vi "Acquire multiple shots.vi"(7 "DAQ":T1={"Data"={"Live"={"t0"=timestamp(0 s since 1904-01-01), "dt"=1.0, "Y"=[]}, "Accumulated"={"t0"=timestamp(0 s since 1904-01-01), "dt"=1.0, "Y"=[]}, "Averaged"={"t0"=timestamp(0 s since 1904-01-01), "dt"=1.0, "Y"=[]}, "data array"=[], "live time array"=[], "Live (decimated)"={"t0"=timestamp(0 s since 1904-01-01), "dt"=1.0, "Y"=[]}}, "Config"={"Input Config"=0, "Card"=enum."USB-6211", "100% Reflectance Standard (V)"=0.0, "Input Channel"="", "Average number of points"=0.0, "Trigger Level (V)"=0.0, "Rate (Hz)"=0, "End Time (s)"=0.0}, "Indicators"={"Final number of points"=0.0, "Number of samples"=0.0, "dt"=0.0, "Shots"=10, "Shot counter"=10, "Test counter"=10, "Background level (V)"=0.0, "DAQ task"="", "timestamp of data"=timestamp(0 s since 1904-01-01), "Test Type"=enum."A-Test"}} {"Config"."Input Config" items=["default"=-1, "RSE"=10083, "NRSE"=10078, "Differential"=10106, "Pseudodifferential"=12529]}, 8 "error in (no error)":errorcluster) -> (0 "error out":errorcluster, 5 "DAQ out":T1={"Data"={"Live"={"t0"=timestamp(0 s since 1904-01-01), "dt"=1.0, "Y"=[]}, "Accumulated"={"t0"=timestamp(0 s since 1904-01-01), "dt"=1.0, "Y"=[]}, "Averaged"={"t0"=timestamp(0 s since 1904-01-01), "dt"=1.0, "Y"=[]}, "data array"=[], "live time array"=[], "Live (decimated)"={"t0"=timestamp(0 s since 1904-01-01), "dt"=1.0, "Y"=[]}}, "Config"={"Input Config"=0, "Card"=enum."USB-6211", "100% Reflectance Standard (V)"=0.0, "Input Channel"="", "Average number of points"=0.0, "Trigger Level (V)"=0.0, "Rate (Hz)"=0, "End Time (s)"=0.0}, "Indicators"={"Final number of points"=0.0, "Number of samples"=0.0, "dt"=0.0, "Shots"=10, "Shot counter"=10, "Test counter"=10, "Background level (V)"=0.0, "DAQ task"="", "timestamp of data"=timestamp(0 s since 1904-01-01), "Test Type"=enum."A-Test"}} {"Config"."Input Config" items=["default"=-1, "RSE"=10083, "NRSE"=10078, "Differential"=10106, "Pseudodifferential"=12529]})   [LabVIEW 2017, in "DAQ.lvlib"]
uses:
  DAQ.lvlib
  Controls/Params.ctl
  Controls/DAQ Config.ctl
  Controls/DAQ Indicators.ctl
  System Control/CTLs/Test Type.ctl
  <vilib>/DAQmx/read.llb/DAQmx Read (Analog Wfm 1Chan NSamp).vi
  <vilib>/DAQmx/miscellaneous.llb/DAQmx Fill In Error Info.vi
  System Control/Main controller.lvlib
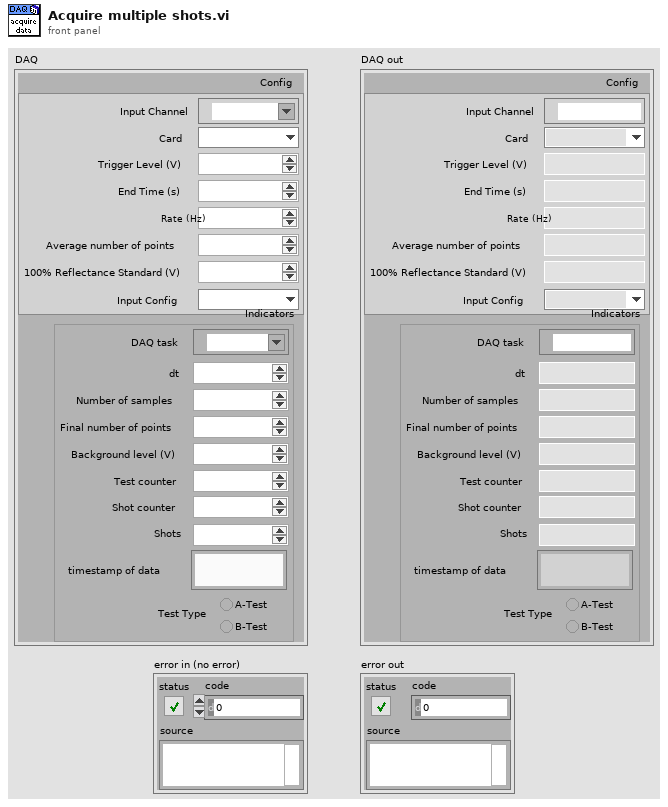
[diagram p1: front panel]
types:
  T1 = typedef "DAQ.lvlib/Params.ctl" = cluster{"Data":cluster{"Live":waveform(dbl), "Accumulated":waveform(dbl), "Averaged":waveform(dbl), "data array":dbl[], "live time array":dbl[], "Live (decimated)":waveform(dbl)}, "Config":T2, "Indicators":T3}
  T2 = typedef "DAQ.lvlib/DAQ Config.ctl" = cluster{"Input Config":i32, "Card":enum16{"USB-6211", "USB-6251", "USB-6361"}, "100% Reflectance Standard (V)":dbl, "Input Channel":tag, "Average number of points":dbl, "Trigger Level (V)":dbl, "Rate (Hz)":i32, "End Time (s)":dbl}
  T3 = typedef "DAQ.lvlib/DAQ Indicators.ctl" = cluster{"Final number of points":dbl, "Number of samples":dbl, "dt":dbl, "Shots":i32, "Shot counter":i32, "Test counter":i32, "Background level (V)":dbl, "DAQ task":refnum<k21>, "timestamp of data":timestamp, "Test Type":T4}
  T4 = typedef "Main controller.lvlib/Test Type.ctl" = enum32{"A-Test", "B-Test"}
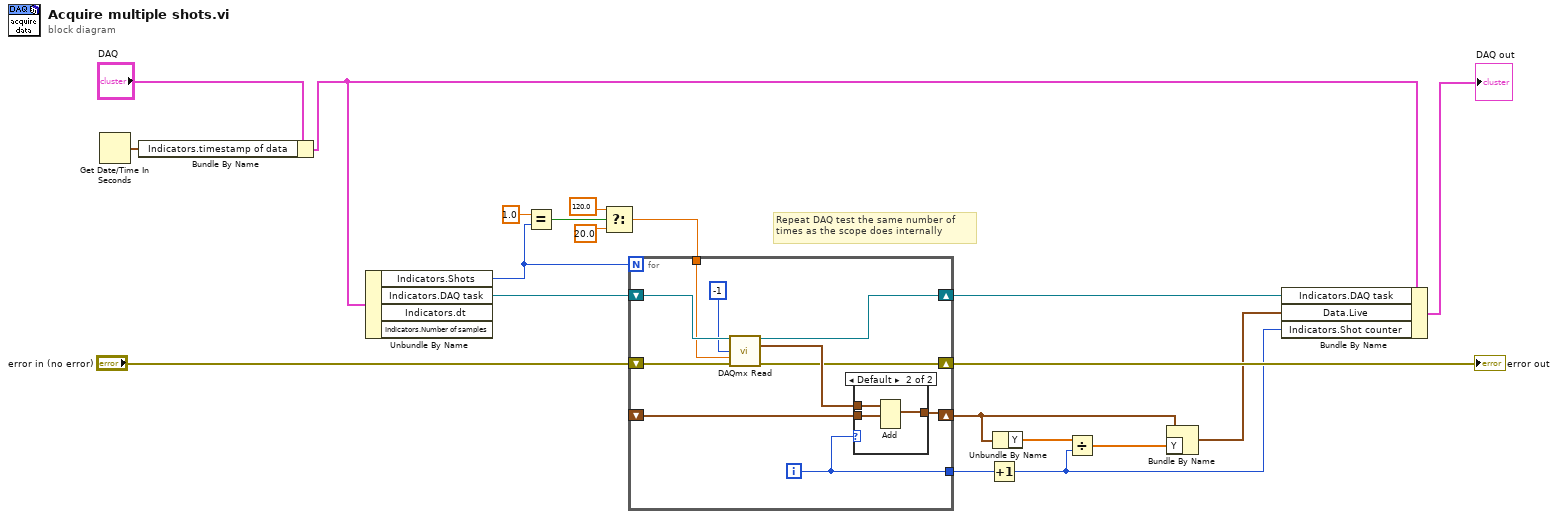
[diagram p0: block diagram]
diagram:
  # "Repeat DAQ test the same number of \ntimes as the scope does internally"
  n1 = Get Date/Time In Seconds() -> (seconds since 1Jan1904=w6:timestamp)
  n2 = Bundle By Name(cluster="DAQ", "Indicators.timestamp of data"=w6) -> (w2:T1)
  n3 = Unbundle By Name(w2) -> ("Indicators.Shots"=w13:i32, "Indicators.DAQ task"=w12:refnum<k21>)  [unwired: 2 out]
  n4 = Equal?(x=1.0 ("y"), y=w13) -> (x = y?=w17:bool)
  n5 = Select(t=120.0 ("timeout"), s=w17, f=20.0 ("timeout")) -> (s? t:f=w14:dbl)
  n6 = for {
    N: w13 -> [_]
    shift-right: [w26] -> w9
    shift-left: _ -> [w30]
    shift-right: [w22] -> w20
    shift-left: "error in (no error)" -> [w28]
    shift-right: [w29] -> w11
    shift-left: w12 -> [w27]
    tunnel: w14 -> [w23]
    tunnel: [w21] -> w8
    i -> [w21]
    n7 = call-poly <vilib>:"DAQmx Read.vi"("task/channels in"=w27, "number of samples per channel"=-1, "timeout"=w23, "error in"=w28) -> ("task out"=w29:refnum<k21>, "data"=w25:waveform(dbl), "error out"=w22:errorcluster)  [unwired: 9 in]
    n8 = case shown="Default" w21 {
      tunnel: w30 -> [_ w34]
      tunnel: [w31 w33] -> w26
      tunnel: w25 -> [w31 w32]
      frame 0 {
      }
      frame Default {
        n9 = Add(1:w34, 2:w32) -> (0:w33:waveform(dbl))  [unwired: 1 in, 1 out]
      }
    }
  }
  "error out" <- w20
  n10 = Increment(x=w8) -> (x+1=w7:i32)
  n11 = Unbundle By Name(w9) -> ("Y"=w3:dbl[])
  n12 = Divide(x=w3, y=w7) -> (x/y=w1:dbl[])
  n13 = Bundle By Name(cluster=w9, "Y"=w1) -> (w4:waveform(dbl))
  n14 = Bundle By Name(cluster=w2, "Indicators.DAQ task"=w11, "Data.Live"=w4, "Indicators.Shot counter"=w7) -> (→"DAQ out":T1)
